vi "python hdf5 example.vi"() -> ()   [LabVIEW 2020]
panel:
  in  "error in (no error)":errorcluster
  out "error out":errorcluster
  in  "hdf5 root path":path=path "C:/GEECS/data"
  in  "image #":i16=1
  in  "camera name":string="Camera1"
  in  "Python version":string="3.8"
  in  "module path":path=path "C:/GEECS/Developers Version/source/Axel/openPMD-CCD/openpmd_ccd_labview.py"
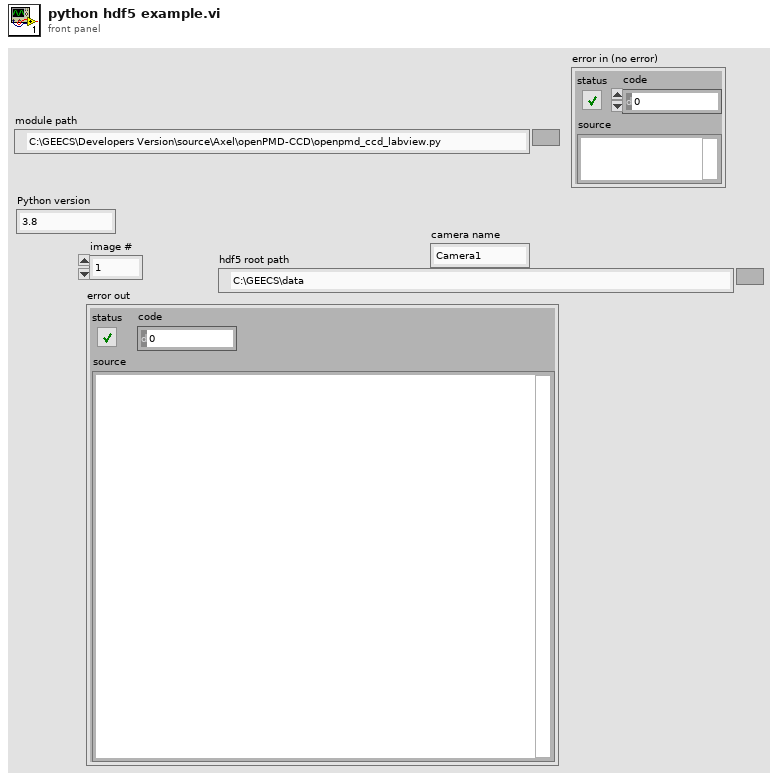
[diagram p1: front panel]
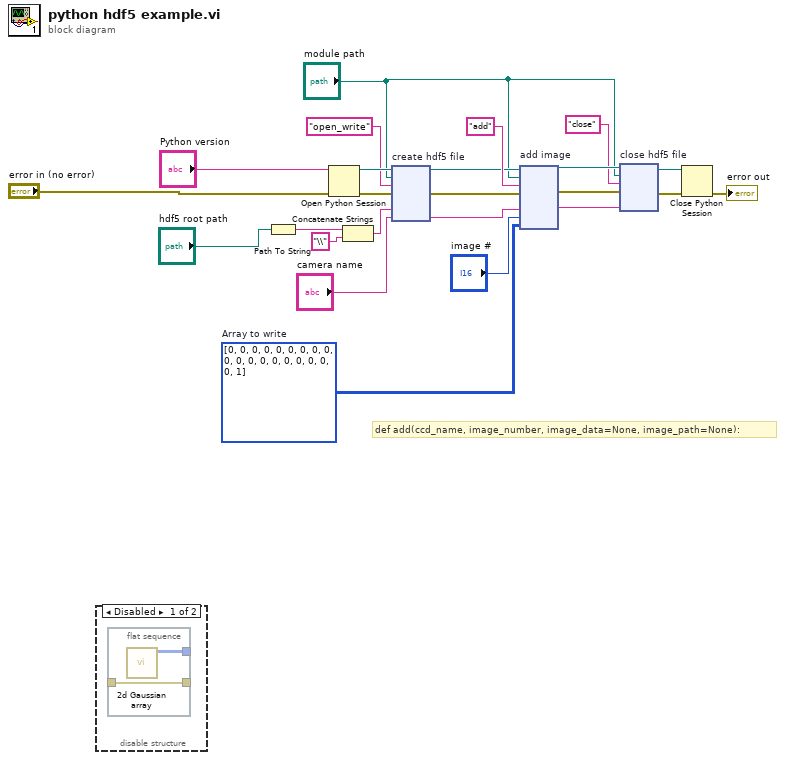
[diagram p0: block diagram]
diagram:
  w3 = u16[][] [[0, 0, 0, 0, 0], [0, 0, 0, 0, 0], [0, 0, 0, 0, 0], [0, 0, 0, 0, 1]]  # Array to write
  # "def add(ccd_name, image_number, image_data=None, image_path=None):"
  n1 = disable-structure shown="Disabled" {
    frame Disabled {
      n2 = flat-sequence {
        tunnel: [w26] -> _
        tunnel: _ -> [w25]
        tunnel: [w25] -> _
        frame #0 {
          n3 = call "2d Gaussian array.vi"() -> ("Intensity Graph"=w26:u16[][])  [unwired: 11 in]
        }
      }
    }
    frame Enabled {
    }
  }
  n4 = Path To String(path="hdf5 root path") -> (string=w15:string)
  n5 = Open Python Session(python version="Python version", 3:"error in (no error)") -> (session out=w22:refnum<k35>, error out=w8:errorcluster)  [unwired: 1 in]
  n6 = Concatenate Strings(w15, "\\") -> (w13:string)
  n7 = node "create hdf5 file"(w22, "module path", "open_write" ("open h5 function"), w8, w13, "camera name") -> (w21:refnum<k35>, w4:errorcluster, w12:string)  [unwired: 3 in, 2 out]
  n8 = node "add image"(w21, "module path", "add" ("function name"), w4, w12, "image #", w3) -> (w20:refnum<k35>, w9:errorcluster, w11:string)  [unwired: 4 in, 2 out]
  n9 = node "close hdf5 file"(w20, "module path", "close" ("function name"), w9, w11) -> (w17:refnum<k35>, w10:errorcluster)  [unwired: 3 in, 2 out]
  n10 = Close Python Session(session in=w17, error in=w10) -> (11:→"error out":errorcluster)
